vi "大富翁.vi"() -> ()   [LabVIEW 2014] (continued)
                        n2318 = property on="11房1" class="Bool (strict)"("Visible"=TRUE) -> ()  [unwired: 2 in, 2 out]
                      }
                    }
                  }
                  frame 2 {
                    n2319 = flat-sequence {
                      frame #0 {
                        n2320 = local write "11房2"(TRUE ("1房2")) -> ()
                      }
                      frame #1 {
                        n2321 = property on="11房2" class="Bool (strict)"("Visible"=TRUE ("1房2")) -> ()  [unwired: 2 in, 2 out]
                      }
                    }
                  }
                  frame 3 {
                    n2322 = flat-sequence {
                      frame #0 {
                        n2323 = local write "11房3"(TRUE) -> ()
                      }
                      frame #1 {
                        n2324 = property on="11房3" class="Bool (strict)"("Visible"=TRUE) -> ()  [unwired: 2 in, 2 out]
                      }
                    }
                  }
                  frame 4 {
                    n2325 = flat-sequence {
                      frame #0 {
                        n2326 = local write "11房4"(TRUE) -> ()
                      }
                      frame #1 {
                        n2327 = property on="11房4" class="Bool (strict)"("Visible"=TRUE) -> ()  [unwired: 2 in, 2 out]
                      }
                    }
                  }
                  frame 5 {
                    n2328 = flat-sequence {
                      frame #0 {
                        n2329 = local write "11旅1"(TRUE) -> ()
                      }
                      frame #1 {
                        n2330 = property on="11旅1" class="Bool (strict)"("Visible"=TRUE) -> ()  [unwired: 2 in, 2 out]
                      }
                    }
                  }
                  frame 6 {
                    n2331 = flat-sequence {
                      frame #0 {
                        n2332 = local write "11旅2"(TRUE) -> ()
                      }
                      frame #1 {
                        n2333 = property on="11旅2" class="Bool (strict)"("Visible"=TRUE) -> ()  [unwired: 2 in, 2 out]
                      }
                    }
                  }
                  frame 7 {
                    n2334 = flat-sequence {
                      frame #0 {
                        n2335 = local write "11旅3"(TRUE) -> ()
                      }
                      frame #1 {
                        n2336 = property on="11旅3" class="Bool (strict)"("Visible"=TRUE) -> ()  [unwired: 2 in, 2 out]
                      }
                    }
                  }
                  frame 8 {
                    n2337 = flat-sequence {
                      frame #0 {
                        n2338 = local write "11旅4"(TRUE) -> ()
                      }
                      frame #1 {
                        n2339 = property on="11旅4" class="Bool (strict)"("Visible"=TRUE) -> ()  [unwired: 2 in, 2 out]
                      }
                    }
                  }
                }
                n2340 = case shown="1, Default" w1722 {
                  tunnel: w1726 -> [w1758 w1759 w1760 w1761]
                  frame 1, Default {
                    n2341 = local write "玩家一財產"(w1758) -> ()
                  }
                  frame 2 {
                    n2342 = local write "玩家二財產"(w1759) -> ()
                  }
                  frame 3 {
                    n2343 = local write "玩家三財產"(w1760) -> ()
                  }
                  frame 4 {
                    n2344 = local write "玩家四財產"(w1761) -> ()
                  }
                }
              }
              frame True {
                # "無主地"
                n2345 = call "購買土地.vi"() -> ("確定 2"=w1768:bool)  [unwired: 3 in]
                n2346 = case shown="True" w1768 {
                  tunnel: w1767 -> [_ w1772]
                  frame False {
                    # "不買"
                  }
                  frame True {
                    # "要買"
                    n2347 = local read "換誰?"() -> (w1773:dbl)
                    n2348 = case shown="4" w1773 {
                      tunnel: [w1800 w1801 w1802 w1803] -> w1771
                      frame 1, Default {
                        n2349 = local read "玩家一財產"() -> (w1800:dbl)
                      }
                      frame 2 {
                        n2350 = local read "玩家二財產"() -> (w1801:dbl)
                      }
                      frame 3 {
                        n2351 = local read "玩家三財產"() -> (w1802:dbl)
                      }
                      frame 4 {
                        n2352 = local read "玩家四財產"() -> (w1803:dbl)
                      }
                    }
                    n2353 = call "各種價格.vi"("Numeric"=w1772) -> ("買空地"=w1770:dbl)  [unwired: 4 in, 5 out]
                    n2354 = Greater Or Equal?(x=w1771, y=w1770) -> (x >= y?=w1769:bool)
                    n2355 = case shown="True" w1769 {
                      tunnel: w1772 -> [_ w1774]
                      frame False {
                        # "錢不夠"
                        n2356 = call "錢不夠.vi"() -> ()  [unwired: 4 in]
                      }
                      frame True {
                        # "錢夠"
                        n2357 = local read "換誰?"() -> (w1775:dbl)
                        n2358 = case shown="2" w1775 {
                          selector: w1775 -> [w1779 w1785 w1791 w1797]
                          tunnel: w1774 -> [w1778 w1784 w1790 w1796]
                          frame 1, Default {
                            # "誰買了地"
                            n2359 = call "各種價格.vi"("Numeric"=w1778) -> ("買空地"=w1777:dbl)  [unwired: 4 in, 5 out]
                            n2360 = local read "玩家一財產"() -> (w1781:dbl)
                            n2361 = Subtract(x=w1781, y=w1777) -> (x-y=w1780:dbl)
                            n2362 = local write "玩家一財產"(w1780) -> ()
                            n2363 = call "數字轉顏色.vi"("數字"=w1779) -> ("顏色數字"=w1776:dbl)  [unwired: 2 in]
                            n2364 = local write "11蘭嶼"(w1776) -> ()
                            n2365 = local write "蘭嶼所有"(w1776) -> ()
                          }
                          frame 2 {
                            # "誰買了地"
                            n2366 = call "各種價格.vi"("Numeric"=w1784) -> ("買空地"=w1783:dbl)  [unwired: 4 in, 5 out]
                            n2367 = local read "玩家二財產"() -> (w1787:dbl)
                            n2368 = Subtract(x=w1787, y=w1783) -> (x-y=w1786:dbl)
                            n2369 = local write "玩家二財產"(w1786) -> ()
                            n2370 = call "數字轉顏色.vi"("數字"=w1785) -> ("顏色數字"=w1782:dbl)  [unwired: 2 in]
                            n2371 = local write "11蘭嶼"(w1782) -> ()
                            n2372 = local write "蘭嶼所有"(w1782) -> ()
                          }
                          frame 3 {
                            # "誰買了地"
                            n2373 = local read "玩家三財產"() -> (w1792:dbl)
                            n2374 = call "各種價格.vi"("Numeric"=w1790) -> ("買空地"=w1789:dbl)  [unwired: 4 in, 5 out]
                            n2375 = Subtract(x=w1792, y=w1789) -> (x-y=w1793:dbl)
                            n2376 = call "數字轉顏色.vi"("數字"=w1791) -> ("顏色數字"=w1788:dbl)  [unwired: 2 in]
                            n2377 = local write "玩家三財產"(w1793) -> ()
                            n2378 = local write "11蘭嶼"(w1788) -> ()
                            n2379 = local write "蘭嶼所有"(w1788) -> ()
                          }
                          frame 4 {
                            # "誰買了地"
                            n2380 = call "各種價格.vi"("Numeric"=w1796) -> ("買空地"=w1795:dbl)  [unwired: 4 in, 5 out]
                            n2381 = local read "玩家四財產"() -> (w1799:dbl)
                            n2382 = Subtract(x=w1799, y=w1795) -> (x-y=w1798:dbl)
                            n2383 = local write "玩家四財產"(w1798) -> ()
                            n2384 = call "數字轉顏色.vi"("數字"=w1797) -> ("顏色數字"=w1794:dbl)  [unwired: 2 in]
                            n2385 = local write "11蘭嶼"(w1794) -> ()
                            n2386 = local write "蘭嶼所有"(w1794) -> ()
                          }
                        }
                      }
                    }
                  }
                }
              }
            }
          }
          frame 12 {
            n2387 = local read "金門縣所有"() -> (w1804:u32)
            n2388 = Equal?(x=w1804, y=u32 16777215) -> (x = y?=w1807:bool)
            n2389 = case shown="False" w1807 {
              tunnel: w1806 -> [w1830 w1868]
              tunnel: [w1820 FALSE] -> w1805
              frame False {
                # "有主地"
                n2390 = local read "換誰?"() -> (w1823:dbl)
                n2391 = local read "金門縣所有"() -> (w1811:u32)
                n2392 = call "數字轉顏色.vi"("數字"=w1823) -> ("顏色數字"=w1834:dbl)  [unwired: 2 in]
                n2393 = case shown="4" w1823 {
                  tunnel: [w1863 w1864 w1865 w1866] -> w1829
                  frame 1, Default {
                    n2394 = local read "玩家一財產"() -> (w1863:dbl)
                  }
                  frame 2 {
                    n2395 = local read "玩家二財產"() -> (w1864:dbl)
                  }
                  frame 3 {
                    n2396 = local read "玩家三財產"() -> (w1865:dbl)
                  }
                  frame 4 {
                    n2397 = local read "玩家四財產"() -> (w1866:dbl)
                  }
                }
                n2398 = Equal?(x=w1811, y=w1834) -> (x = y?=w1833:bool)
                n2399 = local read "12旅4"() -> (w1819:bool)
                n2400 = local read "12旅3"() -> (w1818:bool)
                n2401 = local read "12旅2"() -> (w1817:bool)
                n2402 = local read "12旅1"() -> (w1816:bool)
                n2403 = local read "12房4"() -> (w1815:bool)
                n2404 = local read "12房3"() -> (w1814:bool)
                n2405 = local read "12房2"() -> (w1813:bool)
                n2406 = local read "12房1"() -> (w1812:bool)
                n2407 = local read "金門縣所有"() -> (w1810:u32)
                n2408 = call "房子數量.vi"("房子 1"=w1812, "房子 2"=w1813, "房子 3"=w1814, "房子 4"=w1815, "旅館 1"=w1816, "旅館 2"=w1817, "旅館 3"=w1818, "旅館 4"=w1819) -> ("房子數"=w1832:dbl, "旅館數"=w1831:dbl)  [unwired: 18 in]
                n2409 = call "顏色轉數字.vi"("顏色數字"=w1810) -> ("數字"=w1821:dbl)  [unwired: 2 in]
                n2410 = case shown="1, Default" w1821 {
                  tunnel: [w1839 w1840 w1841 w1842] -> w1825
                  frame 1, Default {
                    n2411 = local read "玩家一財產"() -> (w1839:dbl)
                  }
                  frame 2 {
                    n2412 = local read "玩家二財產"() -> (w1840:dbl)
                  }
                  frame 3 {
                    n2413 = local read "玩家三財產"() -> (w1841:dbl)
                  }
                  frame 4 {
                    n2414 = local read "玩家四財產"() -> (w1842:dbl)
                  }
                }
                n2415 = call "走到地.vi"("房子數量"=w1832, "自己的地?"=w1833, "旅館數量"=w1831, "編號"=w1830, "走到人財產"=w1829) -> ("走到人-?"=w1828:dbl, "蓋第幾棟"=w1826:dbl, "地主+?"=w1824:dbl, "破產?"=w1820:bool)
                n2416 = Subtract(x=w1829, y=w1828) -> (x-y=w1827:dbl)
                n2417 = Add(x=w1824, y=w1825) -> (x+y=w1822:dbl)
                n2418 = case shown="2" w1821 {
                  tunnel: w1822 -> [w1835 w1836 w1837 w1838]
                  frame 1, Default {
                    n2419 = local write "玩家一財產"(w1835) -> ()
                  }
                  frame 2 {
                    n2420 = local write "玩家二財產"(w1836) -> ()
                  }
                  frame 3 {
                    n2421 = local write "玩家三財產"(w1837) -> ()
                  }
                  frame 4 {
                    n2422 = local write "玩家四財產"(w1838) -> ()
                  }
                }
                n2423 = case shown="2" w1826 {
                  frame 0, Default {
                  }
                  frame 1 {
                    n2424 = flat-sequence {
                      frame #0 {
                        n2425 = local write "12房1"(TRUE ("1房1")) -> ()
                      }
                      frame #1 {
                        n2426 = property on="12房1" class="Bool (strict)"("Visible"=TRUE) -> ()  [unwired: 2 in, 2 out]
                      }
                    }
                  }
                  frame 2 {
                    n2427 = flat-sequence {
                      frame #0 {
                        n2428 = local write "12房2"(TRUE ("1房2")) -> ()
                      }
                      frame #1 {
                        n2429 = property on="12房2" class="Bool (strict)"("Visible"=TRUE ("1房2")) -> ()  [unwired: 2 in, 2 out]
                      }
                    }
                  }
                  frame 3 {
                    n2430 = flat-sequence {
                      frame #0 {
                        n2431 = local write "12房3"(TRUE) -> ()
                      }
                      frame #1 {
                        n2432 = property on="12房3" class="Bool (strict)"("Visible"=TRUE) -> ()  [unwired: 2 in, 2 out]
                      }
                    }
                  }
                  frame 4 {
                    n2433 = flat-sequence {
                      frame #0 {
                        n2434 = local write "12房4"(TRUE) -> ()
                      }
                      frame #1 {
                        n2435 = property on="12房4" class="Bool (strict)"("Visible"=TRUE) -> ()  [unwired: 2 in, 2 out]
                      }
                    }
                  }
                  frame 5 {
                    n2436 = flat-sequence {
                      frame #0 {
                        n2437 = local write "12旅1"(TRUE) -> ()
                      }
                      frame #1 {
                        n2438 = property on="12旅1" class="Bool (strict)"("Visible"=TRUE) -> ()  [unwired: 2 in, 2 out]
                      }
                    }
                  }
                  frame 6 {
                    n2439 = flat-sequence {
                      frame #0 {
                        n2440 = local write "12旅2"(TRUE) -> ()
                      }
                      frame #1 {
                        n2441 = property on="12旅2" class="Bool (strict)"("Visible"=TRUE) -> ()  [unwired: 2 in, 2 out]
                      }
                    }
                  }
                  frame 7 {
                    n2442 = flat-sequence {
                      frame #0 {
                        n2443 = local write "12旅3"(TRUE) -> ()
                      }
                      frame #1 {
                        n2444 = property on="12旅3" class="Bool (strict)"("Visible"=TRUE) -> ()  [unwired: 2 in, 2 out]
                      }
                    }
                  }
                  frame 8 {
                    n2445 = flat-sequence {
                      frame #0 {
                        n2446 = local write "12旅4"(TRUE) -> ()
                      }
                      frame #1 {
                        n2447 = property on="12旅4" class="Bool (strict)"("Visible"=TRUE) -> ()  [unwired: 2 in, 2 out]
                      }
                    }
                  }
                }
                n2448 = case shown="1, Default" w1823 {
                  tunnel: w1827 -> [w1859 w1860 w1861 w1862]
                  frame 1, Default {
                    n2449 = local write "玩家一財產"(w1859) -> ()
                  }
                  frame 2 {
                    n2450 = local write "玩家二財產"(w1860) -> ()
                  }
                  frame 3 {
                    n2451 = local write "玩家三財產"(w1861) -> ()
                  }
                  frame 4 {
                    n2452 = local write "玩家四財產"(w1862) -> ()
                  }
                }
              }
              frame True {
                # "無主地"
                n2453 = call "購買土地.vi"() -> ("確定 2"=w1869:bool)  [unwired: 3 in]
                n2454 = case shown="True" w1869 {
                  tunnel: w1868 -> [_ w1873]
                  frame False {
                    # "不買"
                  }
                  frame True {
                    # "要買"
                    n2455 = local read "換誰?"() -> (w1874:dbl)
                    n2456 = case shown="4" w1874 {
                      tunnel: [w1901 w1902 w1903 w1904] -> w1872
                      frame 1, Default {
                        n2457 = local read "玩家一財產"() -> (w1901:dbl)
                      }
                      frame 2 {
                        n2458 = local read "玩家二財產"() -> (w1902:dbl)
                      }
                      frame 3 {
                        n2459 = local read "玩家三財產"() -> (w1903:dbl)
                      }
                      frame 4 {
                        n2460 = local read "玩家四財產"() -> (w1904:dbl)
                      }
                    }
                    n2461 = call "各種價格.vi"("Numeric"=w1873) -> ("買空地"=w1871:dbl)  [unwired: 4 in, 5 out]
                    n2462 = Greater Or Equal?(x=w1872, y=w1871) -> (x >= y?=w1870:bool)
                    n2463 = case shown="True" w1870 {
                      tunnel: w1873 -> [_ w1875]
                      frame False {
                        # "錢不夠"
                        n2464 = call "錢不夠.vi"() -> ()  [unwired: 4 in]
                      }
                      frame True {
                        # "錢夠"
                        n2465 = local read "換誰?"() -> (w1876:dbl)
                        n2466 = case shown="1, Default" w1876 {
                          selector: w1876 -> [w1880 w1886 w1892 w1898]
                          tunnel: w1875 -> [w1879 w1885 w1891 w1897]
                          frame 1, Default {
                            # "誰買了地"
                            n2467 = call "各種價格.vi"("Numeric"=w1879) -> ("買空地"=w1878:dbl)  [unwired: 4 in, 5 out]
                            n2468 = local read "玩家一財產"() -> (w1882:dbl)
                            n2469 = Subtract(x=w1882, y=w1878) -> (x-y=w1881:dbl)
                            n2470 = local write "玩家一財產"(w1881) -> ()
                            n2471 = call "數字轉顏色.vi"("數字"=w1880) -> ("顏色數字"=w1877:dbl)  [unwired: 2 in]
                            n2472 = local write "12金門"(w1877) -> ()
                            n2473 = local write "金門縣所有"(w1877) -> ()
                          }
                          frame 2 {
                            # "誰買了地"
                            n2474 = call "各種價格.vi"("Numeric"=w1885) -> ("買空地"=w1884:dbl)  [unwired: 4 in, 5 out]
                            n2475 = local read "玩家二財產"() -> (w1888:dbl)
                            n2476 = Subtract(x=w1888, y=w1884) -> (x-y=w1887:dbl)
                            n2477 = local write "玩家二財產"(w1887) -> ()
                            n2478 = call "數字轉顏色.vi"("數字"=w1886) -> ("顏色數字"=w1883:dbl)  [unwired: 2 in]
                            n2479 = local write "12金門"(w1883) -> ()
                            n2480 = local write "金門縣所有"(w1883) -> ()
                          }
                          frame 3 {
                            # "誰買了地"
                            n2481 = local read "玩家三財產"() -> (w1893:dbl)
                            n2482 = call "各種價格.vi"("Numeric"=w1891) -> ("買空地"=w1890:dbl)  [unwired: 4 in, 5 out]
                            n2483 = Subtract(x=w1893, y=w1890) -> (x-y=w1894:dbl)
                            n2484 = call "數字轉顏色.vi"("數字"=w1892) -> ("顏色數字"=w1889:dbl)  [unwired: 2 in]
                            n2485 = local write "玩家三財產"(w1894) -> ()
                            n2486 = local write "12金門"(w1889) -> ()
                            n2487 = local write "金門縣所有"(w1889) -> ()
                          }
                          frame 4 {
                            # "誰買了地"
                            n2488 = call "各種價格.vi"("Numeric"=w1897) -> ("買空地"=w1896:dbl)  [unwired: 4 in, 5 out]
                            n2489 = local read "玩家四財產"() -> (w1900:dbl)
                            n2490 = Subtract(x=w1900, y=w1896) -> (x-y=w1899:dbl)
                            n2491 = local write "玩家四財產"(w1899) -> ()
                            n2492 = call "數字轉顏色.vi"("數字"=w1898) -> ("顏色數字"=w1895:dbl)  [unwired: 2 in]
                            n2493 = local write "12金門"(w1895) -> ()
                            n2494 = local write "金門縣所有"(w1895) -> ()
                          }
                        }
                      }
                    }
                  }
                }
              }
            }
          }
          frame 13 {
            n2495 = call "13監獄.vi"() -> ()  [unwired: 4 in]
          }
          frame 14 {
            n2496 = local read "馬祖所有"() -> (w1907:u32)
            n2497 = Equal?(x=w1907, y=u32 16777215) -> (x = y?=w1910:bool)
            n2498 = case shown="False" w1910 {
              tunnel: w1909 -> [w1933 w1971]
              tunnel: [w1923 FALSE] -> w1908
              frame False {
                # "有主地"
                n2499 = local read "馬祖所有"() -> (w1913:u32)
                n2500 = local read "換誰?"() -> (w1926:dbl)
                n2501 = call "數字轉顏色.vi"("數字"=w1926) -> ("顏色數字"=w1937:dbl)  [unwired: 2 in]
                n2502 = case shown="4" w1926 {
                  tunnel: [w1966 w1967 w1968 w1969] -> w1932
                  frame 1, Default {
                    n2503 = local read "玩家一財產"() -> (w1966:dbl)
                  }
                  frame 2 {
                    n2504 = local read "玩家二財產"() -> (w1967:dbl)
                  }
                  frame 3 {
                    n2505 = local read "玩家三財產"() -> (w1968:dbl)
                  }
                  frame 4 {
                    n2506 = local read "玩家四財產"() -> (w1969:dbl)
                  }
                }
                n2507 = Equal?(x=w1913, y=w1937) -> (x = y?=w1936:bool)
                n2508 = local read "馬祖所有"() -> (w1914:u32)
                n2509 = local read "14旅4"() -> (w1915:bool)
                n2510 = local read "14旅3"() -> (w1916:bool)
                n2511 = local read "14旅2"() -> (w1917:bool)
                n2512 = local read "14旅1"() -> (w1918:bool)
                n2513 = local read "14房4"() -> (w1919:bool)
                n2514 = local read "14房3"() -> (w1920:bool)
                n2515 = local read "14房2"() -> (w1921:bool)
                n2516 = local read "14房1"() -> (w1922:bool)
                n2517 = call "房子數量.vi"("房子 1"=w1922, "房子 2"=w1921, "房子 3"=w1920, "房子 4"=w1919, "旅館 1"=w1918, "旅館 2"=w1917, "旅館 3"=w1916, "旅館 4"=w1915) -> ("房子數"=w1935:dbl, "旅館數"=w1934:dbl)  [unwired: 18 in]
                n2518 = call "顏色轉數字.vi"("顏色數字"=w1914) -> ("數字"=w1924:dbl)  [unwired: 2 in]
                n2519 = case shown="1, Default" w1924 {
                  tunnel: [w1942 w1943 w1944 w1945] -> w1928
                  frame 1, Default {
                    n2520 = local read "玩家一財產"() -> (w1942:dbl)
                  }
                  frame 2 {
                    n2521 = local read "玩家二財產"() -> (w1943:dbl)
                  }
                  frame 3 {
                    n2522 = local read "玩家三財產"() -> (w1944:dbl)
                  }
                  frame 4 {
                    n2523 = local read "玩家四財產"() -> (w1945:dbl)
                  }
                }
                n2524 = call "走到地.vi"("房子數量"=w1935, "自己的地?"=w1936, "旅館數量"=w1934, "編號"=w1933, "走到人財產"=w1932) -> ("走到人-?"=w1931:dbl, "蓋第幾棟"=w1929:dbl, "地主+?"=w1927:dbl, "破產?"=w1923:bool)
                n2525 = Subtract(x=w1932, y=w1931) -> (x-y=w1930:dbl)
                n2526 = Add(x=w1927, y=w1928) -> (x+y=w1925:dbl)
                n2527 = case shown="1, Default" w1924 {
                  tunnel: w1925 -> [w1938 w1939 w1940 w1941]
                  frame 1, Default {
                    n2528 = local write "玩家一財產"(w1938) -> ()
                  }
                  frame 2 {
                    n2529 = local write "玩家二財產"(w1939) -> ()
                  }
                  frame 3 {
                    n2530 = local write "玩家三財產"(w1940) -> ()
                  }
                  frame 4 {
                    n2531 = local write "玩家四財產"(w1941) -> ()
                  }
                }
                n2532 = case shown="8" w1929 {
                  frame 0, Default {
                  }
                  frame 1 {
                    n2533 = flat-sequence {
                      frame #0 {
                        n2534 = local write "14房1"(TRUE ("1房1")) -> ()
                      }
                      frame #1 {
                        n2535 = property on="14房1" class="Bool (strict)"("Visible"=TRUE) -> ()  [unwired: 2 in, 2 out]
                      }
                    }
                  }
                  frame 2 {
                    n2536 = flat-sequence {
                      frame #0 {
                        n2537 = local write "14房2"(TRUE ("1房2")) -> ()
                      }
                      frame #1 {
                        n2538 = property on="14房2" class="Bool (strict)"("Visible"=TRUE ("1房2")) -> ()  [unwired: 2 in, 2 out]
                      }
                    }
                  }
                  frame 3 {
                    n2539 = flat-sequence {
                      frame #0 {
                        n2540 = local write "14房3"(TRUE) -> ()
                      }
                      frame #1 {
                        n2541 = property on="14房3" class="Bool (strict)"("Visible"=TRUE) -> ()  [unwired: 2 in, 2 out]
                      }
                    }
                  }
                  frame 4 {
                    n2542 = flat-sequence {
                      frame #0 {
                        n2543 = local write "14房4"(TRUE) -> ()
                      }
                      frame #1 {
                        n2544 = property on="14房4" class="Bool (strict)"("Visible"=TRUE) -> ()  [unwired: 2 in, 2 out]
                      }
                    }
                  }
                  frame 5 {
                    n2545 = flat-sequence {
                      frame #0 {
                        n2546 = local write "14旅1"(TRUE) -> ()
                      }
                      frame #1 {
                        n2547 = property on="14旅1" class="Bool (strict)"("Visible"=TRUE) -> ()  [unwired: 2 in, 2 out]
                      }
                    }
                  }
                  frame 6 {
                    n2548 = flat-sequence {
                      frame #0 {
                        n2549 = local write "14旅2"(TRUE) -> ()
                      }
                      frame #1 {
                        n2550 = property on="14旅2" class="Bool (strict)"("Visible"=TRUE) -> ()  [unwired: 2 in, 2 out]
                      }
                    }
                  }
                  frame 7 {
                    n2551 = flat-sequence {
                      frame #0 {
                        n2552 = local write "14旅3"(TRUE) -> ()
                      }
                      frame #1 {
                        n2553 = property on="14旅3" class="Bool (strict)"("Visible"=TRUE) -> ()  [unwired: 2 in, 2 out]
                      }
                    }
                  }
                  frame 8 {
                    n2554 = flat-sequence {
                      frame #0 {
                        n2555 = local write "14旅4"(TRUE) -> ()
                      }
                      frame #1 {
                        n2556 = property on="14旅4" class="Bool (strict)"("Visible"=TRUE) -> ()  [unwired: 2 in, 2 out]
                      }
                    }
                  }
                }
                n2557 = case shown="1, Default" w1926 {
                  tunnel: w1930 -> [w1962 w1963 w1964 w1965]
                  frame 1, Default {
                    n2558 = local write "玩家一財產"(w1962) -> ()
                  }
                  frame 2 {
                    n2559 = local write "玩家二財產"(w1963) -> ()
                  }
                  frame 3 {
                    n2560 = local write "玩家三財產"(w1964) -> ()
                  }
                  frame 4 {
                    n2561 = local write "玩家四財產"(w1965) -> ()
                  }
                }
              }
              frame True {
                # "無主地"
                n2562 = call "購買土地.vi"() -> ("確定 2"=w1972:bool)  [unwired: 3 in]
                n2563 = case shown="True" w1972 {
                  tunnel: w1971 -> [_ w1976]
                  frame False {
                    # "不買"
                  }
                  frame True {
                    # "要買"
                    n2564 = local read "換誰?"() -> (w1977:dbl)
                    n2565 = case shown="4" w1977 {
                      tunnel: [w2004 w2005 w2006 w2007] -> w1975
                      frame 1, Default {
                        n2566 = local read "玩家一財產"() -> (w2004:dbl)
                      }
                      frame 2 {
                        n2567 = local read "玩家二財產"() -> (w2005:dbl)
                      }
                      frame 3 {
                        n2568 = local read "玩家三財產"() -> (w2006:dbl)
                      }
                      frame 4 {
                        n2569 = local read "玩家四財產"() -> (w2007:dbl)
                      }
                    }
                    n2570 = call "各種價格.vi"("Numeric"=w1976) -> ("買空地"=w1974:dbl)  [unwired: 4 in, 5 out]
                    n2571 = Greater Or Equal?(x=w1975, y=w1974) -> (x >= y?=w1973:bool)
                    n2572 = case shown="True" w1973 {
                      tunnel: w1976 -> [_ w1978]
                      frame False {
                        # "錢不夠"
                        n2573 = call "錢不夠.vi"() -> ()  [unwired: 4 in]
                      }
                      frame True {
                        # "錢夠"
                        n2574 = local read "換誰?"() -> (w1979:dbl)
                        n2575 = case shown="2" w1979 {
                          selector: w1979 -> [w1983 w1989 w1995 w2001]
                          tunnel: w1978 -> [w1982 w1988 w1994 w2000]
                          frame 1, Default {
                            # "誰買了地"
                            n2576 = call "各種價格.vi"("Numeric"=w1982) -> ("買空地"=w1981:dbl)  [unwired: 4 in, 5 out]
                            n2577 = local read "玩家一財產"() -> (w1985:dbl)
                            n2578 = Subtract(x=w1985, y=w1981) -> (x-y=w1984:dbl)
                            n2579 = local write "玩家一財產"(w1984) -> ()
                            n2580 = call "數字轉顏色.vi"("數字"=w1983) -> ("顏色數字"=w1980:dbl)  [unwired: 2 in]
                            n2581 = local write "馬祖所有"(w1980) -> ()
                            n2582 = local write "14馬祖"(w1980) -> ()
                          }
                          frame 2 {
                            # "誰買了地"
                            n2583 = call "各種價格.vi"("Numeric"=w1988) -> ("買空地"=w1987:dbl)  [unwired: 4 in, 5 out]
                            n2584 = local read "玩家二財產"() -> (w1991:dbl)
                            n2585 = Subtract(x=w1991, y=w1987) -> (x-y=w1990:dbl)
                            n2586 = local write "玩家二財產"(w1990) -> ()
                            n2587 = call "數字轉顏色.vi"("數字"=w1989) -> ("顏色數字"=w1986:dbl)  [unwired: 2 in]
                            n2588 = local write "馬祖所有"(w1986) -> ()
                            n2589 = local write "14馬祖"(w1986) -> ()
                          }
                          frame 3 {
                            # "誰買了地"
                            n2590 = local read "玩家三財產"() -> (w1996:dbl)
                            n2591 = call "各種價格.vi"("Numeric"=w1994) -> ("買空地"=w1993:dbl)  [unwired: 4 in, 5 out]
                            n2592 = Subtract(x=w1996, y=w1993) -> (x-y=w1997:dbl)
                            n2593 = call "數字轉顏色.vi"("數字"=w1995) -> ("顏色數字"=w1992:dbl)  [unwired: 2 in]
                            n2594 = local write "玩家三財產"(w1997) -> ()
                            n2595 = local write "馬祖所有"(w1992) -> ()
                            n2596 = local write "14馬祖"(w1992) -> ()
                          }
                          frame 4 {
                            # "誰買了地"
                            n2597 = call "各種價格.vi"("Numeric"=w2000) -> ("買空地"=w1999:dbl)  [unwired: 4 in, 5 out]
                            n2598 = local read "玩家四財產"() -> (w2003:dbl)
                            n2599 = Subtract(x=w2003, y=w1999) -> (x-y=w2002:dbl)
                            n2600 = local write "玩家四財產"(w2002) -> ()
                            n2601 = call "數字轉顏色.vi"("數字"=w2001) -> ("顏色數字"=w1998:dbl)  [unwired: 2 in]
                            n2602 = local write "馬祖所有"(w1998) -> ()
                            n2603 = local write "14馬祖"(w1998) -> ()
                          }
                        }
                      }
                    }
                  }
                }
              }
            }
          }
          frame 15 {
            n2604 = local read "小琉球所有"() -> (w2008:u32)
            n2605 = Equal?(x=w2008, y=u32 16777215) -> (x = y?=w2011:bool)
            n2606 = case shown="False" w2011 {
              tunnel: w2009 -> [w2034 w2072]
              tunnel: [w2024 FALSE] -> w2010
              frame False {
                # "有主地"
                n2607 = local read "換誰?"() -> (w2027:dbl)
                n2608 = local read "小琉球所有"() -> (w2015:u32)
                n2609 = call "數字轉顏色.vi"("數字"=w2027) -> ("顏色數字"=w2038:dbl)  [unwired: 2 in]
                n2610 = local read "小琉球所有"() -> (w2014:u32)
                n2611 = case shown="3" w2027 {
                  tunnel: [w2067 w2068 w2069 w2070] -> w2033
                  frame 1, Default {
                    n2612 = local read "玩家一財產"() -> (w2067:dbl)
                  }
                  frame 2 {
                    n2613 = local read "玩家二財產"() -> (w2068:dbl)
                  }
                  frame 3 {
                    n2614 = local read "玩家三財產"() -> (w2069:dbl)
                  }
                  frame 4 {
                    n2615 = local read "玩家四財產"() -> (w2070:dbl)
                  }
                }
                n2616 = Equal?(x=w2015, y=w2038) -> (x = y?=w2037:bool)
                n2617 = local read "15旅4"() -> (w2016:bool)
                n2618 = local read "15旅3"() -> (w2017:bool)
                n2619 = local read "15旅2"() -> (w2018:bool)
                n2620 = local read "15旅1"() -> (w2019:bool)
                n2621 = local read "15房4"() -> (w2020:bool)
                n2622 = local read "15房3"() -> (w2021:bool)
                n2623 = local read "15房2"() -> (w2022:bool)
                n2624 = local read "15房1"() -> (w2023:bool)
                n2625 = call "房子數量.vi"("房子 1"=w2023, "房子 2"=w2022, "房子 3"=w2021, "房子 4"=w2020, "旅館 1"=w2019, "旅館 2"=w2018, "旅館 3"=w2017, "旅館 4"=w2016) -> ("房子數"=w2036:dbl, "旅館數"=w2035:dbl)  [unwired: 18 in]
                n2626 = call "顏色轉數字.vi"("顏色數字"=w2014) -> ("數字"=w2025:dbl)  [unwired: 2 in]
                n2627 = case shown="1, Default" w2025 {
                  tunnel: [w2043 w2044 w2045 w2046] -> w2029
                  frame 1, Default {
                    n2628 = local read "玩家一財產"() -> (w2043:dbl)
                  }
                  frame 2 {
                    n2629 = local read "玩家二財產"() -> (w2044:dbl)
                  }
                  frame 3 {
                    n2630 = local read "玩家三財產"() -> (w2045:dbl)
                  }
                  frame 4 {
                    n2631 = local read "玩家四財產"() -> (w2046:dbl)
                  }
                }
                n2632 = call "走到地.vi"("房子數量"=w2036, "自己的地?"=w2037, "旅館數量"=w2035, "編號"=w2034, "走到人財產"=w2033) -> ("走到人-?"=w2032:dbl, "蓋第幾棟"=w2030:dbl, "地主+?"=w2028:dbl, "破產?"=w2024:bool)
                n2633 = Subtract(x=w2033, y=w2032) -> (x-y=w2031:dbl)
                n2634 = Add(x=w2028, y=w2029) -> (x+y=w2026:dbl)
                n2635 = case shown="1, Default" w2025 {
                  tunnel: w2026 -> [w2039 w2040 w2041 w2042]
                  frame 1, Default {
                    n2636 = local write "玩家一財產"(w2039) -> ()
                  }
                  frame 2 {
                    n2637 = local write "玩家二財產"(w2040) -> ()
                  }
                  frame 3 {
                    n2638 = local write "玩家三財產"(w2041) -> ()
                  }
                  frame 4 {
                    n2639 = local write "玩家四財產"(w2042) -> ()
                  }
                }
                n2640 = case shown="8" w2030 {
                  frame 0, Default {
                  }
                  frame 1 {
                    n2641 = flat-sequence {
                      frame #0 {
                        n2642 = local write "15房1"(TRUE ("1房1")) -> ()
                      }
                      frame #1 {
                        n2643 = property on="15房1" class="Bool (strict)"("Visible"=TRUE) -> ()  [unwired: 2 in, 2 out]
                      }
                    }
                  }
                  frame 2 {
                    n2644 = flat-sequence {
                      frame #0 {
                        n2645 = local write "15房2"(TRUE ("1房2")) -> ()
                      }
                      frame #1 {
                        n2646 = property on="15房2" class="Bool (strict)"("Visible"=TRUE ("1房2")) -> ()  [unwired: 2 in, 2 out]
                      }
                    }
                  }
                  frame 3 {
                    n2647 = flat-sequence {
                      frame #0 {
                        n2648 = local write "15房3"(TRUE) -> ()
                      }
                      frame #1 {
                        n2649 = property on="15房3" class="Bool (strict)"("Visible"=TRUE) -> ()  [unwired: 2 in, 2 out]
                      }
                    }
                  }
                  frame 4 {
                    n2650 = flat-sequence {
                      frame #0 {
                        n2651 = local write "15房4"(TRUE) -> ()
                      }
                      frame #1 {
                        n2652 = property on="15房4" class="Bool (strict)"("Visible"=TRUE) -> ()  [unwired: 2 in, 2 out]
                      }
                    }
                  }
                  frame 5 {
                    n2653 = flat-sequence {
                      frame #0 {
                        n2654 = local write "15旅1"(TRUE) -> ()
                      }
                      frame #1 {
                        n2655 = property on="15旅1" class="Bool (strict)"("Visible"=TRUE) -> ()  [unwired: 2 in, 2 out]
                      }
                    }
                  }
                  frame 6 {
                    n2656 = flat-sequence {
                      frame #0 {
                        n2657 = local write "15旅2"(TRUE) -> ()
                      }
                      frame #1 {
                        n2658 = property on="15旅2" class="Bool (strict)"("Visible"=TRUE) -> ()  [unwired: 2 in, 2 out]
                      }
                    }
                  }
                  frame 7 {
                    n2659 = flat-sequence {
                      frame #0 {
                        n2660 = local write "15旅3"(TRUE) -> ()
                      }
                      frame #1 {
                        n2661 = property on="15旅3" class="Bool (strict)"("Visible"=TRUE) -> ()  [unwired: 2 in, 2 out]
                      }
                    }
                  }
                  frame 8 {
                    n2662 = flat-sequence {
                      frame #0 {
                        n2663 = local write "15旅4"(TRUE) -> ()
                      }
                      frame #1 {
                        n2664 = property on="15旅4" class="Bool (strict)"("Visible"=TRUE) -> ()  [unwired: 2 in, 2 out]
                      }
                    }
                  }
                }
                n2665 = case shown="2" w2027 {
                  tunnel: w2031 -> [w2063 w2064 w2065 w2066]
                  frame 1, Default {
                    n2666 = local write "玩家一財產"(w2063) -> ()
                  }
                  frame 2 {
                    n2667 = local write "玩家二財產"(w2064) -> ()
                  }
                  frame 3 {
                    n2668 = local write "玩家三財產"(w2065) -> ()
                  }
                  frame 4 {
                    n2669 = local write "玩家四財產"(w2066) -> ()
                  }
                }
              }
              frame True {
                # "無主地"
                n2670 = call "購買土地.vi"() -> ("確定 2"=w2073:bool)  [unwired: 3 in]
                n2671 = case shown="True" w2073 {
                  tunnel: w2072 -> [_ w2077]
                  frame False {
                    # "不買"
                  }
                  frame True {
                    # "要買"
                    n2672 = local read "換誰?"() -> (w2078:dbl)
                    n2673 = case shown="4" w2078 {
                      tunnel: [w2105 w2106 w2107 w2108] -> w2076
                      frame 1, Default {
                        n2674 = local read "玩家一財產"() -> (w2105:dbl)
                      }
                      frame 2 {
                        n2675 = local read "玩家二財產"() -> (w2106:dbl)
                      }
                      frame 3 {
                        n2676 = local read "玩家三財產"() -> (w2107:dbl)
                      }
                      frame 4 {
                        n2677 = local read "玩家四財產"() -> (w2108:dbl)
                      }
                    }
                    n2678 = call "各種價格.vi"("Numeric"=w2077) -> ("買空地"=w2075:dbl)  [unwired: 4 in, 5 out]
                    n2679 = Greater Or Equal?(x=w2076, y=w2075) -> (x >= y?=w2074:bool)
                    n2680 = case shown="True" w2074 {
                      tunnel: w2077 -> [_ w2079]
                      frame False {
                        # "錢不夠"
                        n2681 = call "錢不夠.vi"() -> ()  [unwired: 4 in]
                      }
                      frame True {
                        # "錢夠"
                        n2682 = local read "換誰?"() -> (w2080:dbl)
                        n2683 = case shown="1, Default" w2080 {
                          selector: w2080 -> [w2084 w2090 w2096 w2102]
                          tunnel: w2079 -> [w2083 w2089 w2095 w2101]
                          frame 1, Default {
                            # "誰買了地"
                            n2684 = call "各種價格.vi"("Numeric"=w2083) -> ("買空地"=w2082:dbl)  [unwired: 4 in, 5 out]
                            n2685 = local read "玩家一財產"() -> (w2086:dbl)
                            n2686 = Subtract(x=w2086, y=w2082) -> (x-y=w2085:dbl)
                            n2687 = local write "玩家一財產"(w2085) -> ()
                            n2688 = call "數字轉顏色.vi"("數字"=w2084) -> ("顏色數字"=w2081:dbl)  [unwired: 2 in]
                            n2689 = local write "15小琉球"(w2081) -> ()
                            n2690 = local write "小琉球所有"(w2081) -> ()
                          }
                          frame 2 {
                            # "誰買了地"
                            n2691 = call "各種價格.vi"("Numeric"=w2089) -> ("買空地"=w2088:dbl)  [unwired: 4 in, 5 out]
                            n2692 = local read "玩家二財產"() -> (w2092:dbl)
                            n2693 = Subtract(x=w2092, y=w2088) -> (x-y=w2091:dbl)
                            n2694 = local write "玩家二財產"(w2091) -> ()
                            n2695 = call "數字轉顏色.vi"("數字"=w2090) -> ("顏色數字"=w2087:dbl)  [unwired: 2 in]
                            n2696 = local write "15小琉球"(w2087) -> ()
                            n2697 = local write "小琉球所有"(w2087) -> ()
                          }
                          frame 3 {
                            # "誰買了地"
                            n2698 = local read "玩家三財產"() -> (w2097:dbl)
                            n2699 = call "各種價格.vi"("Numeric"=w2095) -> ("買空地"=w2094:dbl)  [unwired: 4 in, 5 out]
                            n2700 = Subtract(x=w2097, y=w2094) -> (x-y=w2098:dbl)
                            n2701 = call "數字轉顏色.vi"("數字"=w2096) -> ("顏色數字"=w2093:dbl)  [unwired: 2 in]
                            n2702 = local write "玩家三財產"(w2098) -> ()
                            n2703 = local write "15小琉球"(w2093) -> ()
                            n2704 = local write "小琉球所有"(w2093) -> ()
                          }
                          frame 4 {
                            # "誰買了地"
                            n2705 = call "各種價格.vi"("Numeric"=w2101) -> ("買空地"=w2100:dbl)  [unwired: 4 in, 5 out]
                            n2706 = local read "玩家四財產"() -> (w2104:dbl)
                            n2707 = Subtract(x=w2104, y=w2100) -> (x-y=w2103:dbl)
                            n2708 = local write "玩家四財產"(w2103) -> ()
                            n2709 = call "數字轉顏色.vi"("數字"=w2102) -> ("顏色數字"=w2099:dbl)  [unwired: 2 in]
                            n2710 = local write "15小琉球"(w2099) -> ()
                            n2711 = local write "小琉球所有"(w2099) -> ()
                          }
                        }
                      }
                    }
                  }
                }
              }
            }
          }
          frame 17 {
            n2712 = local read "墾丁所有"() -> (w2109:u32)
            n2713 = Equal?(x=w2109, y=u32 16777215) -> (x = y?=w2112:bool)
            n2714 = case shown="False" w2112 {
              tunnel: w2110 -> [w2135 w2173]
              tunnel: [w2125 FALSE] -> w2111
              frame False {
                # "有主地"
                n2715 = local read "換誰?"() -> (w2128:dbl)
                n2716 = local read "墾丁所有"() -> (w2116:u32)
                n2717 = call "數字轉顏色.vi"("數字"=w2128) -> ("顏色數字"=w2139:dbl)  [unwired: 2 in]
                n2718 = case shown="4" w2128 {
                  tunnel: [w2168 w2169 w2170 w2171] -> w2134
                  frame 1, Default {
                    n2719 = local read "玩家一財產"() -> (w2168:dbl)
                  }
                  frame 2 {
                    n2720 = local read "玩家二財產"() -> (w2169:dbl)
                  }
                  frame 3 {
                    n2721 = local read "玩家三財產"() -> (w2170:dbl)
                  }
                  frame 4 {
                    n2722 = local read "玩家四財產"() -> (w2171:dbl)
                  }
                }
                n2723 = Equal?(x=w2116, y=w2139) -> (x = y?=w2138:bool)
                n2724 = local read "墾丁所有"() -> (w2115:u32)
                n2725 = local read "17旅4"() -> (w2117:bool)
                n2726 = local read "17旅3"() -> (w2118:bool)
                n2727 = local read "17旅2"() -> (w2119:bool)
                n2728 = local read "17旅1"() -> (w2120:bool)
                n2729 = local read "17房4"() -> (w2121:bool)
                n2730 = local read "17房3"() -> (w2122:bool)
                n2731 = local read "17房2"() -> (w2123:bool)
                n2732 = local read "17房1"() -> (w2124:bool)
                n2733 = call "房子數量.vi"("房子 1"=w2124, "房子 2"=w2123, "房子 3"=w2122, "房子 4"=w2121, "旅館 1"=w2120, "旅館 2"=w2119, "旅館 3"=w2118, "旅館 4"=w2117) -> ("房子數"=w2137:dbl, "旅館數"=w2136:dbl)  [unwired: 18 in]
                n2734 = call "顏色轉數字.vi"("顏色數字"=w2115) -> ("數字"=w2126:dbl)  [unwired: 2 in]
                n2735 = case shown="1, Default" w2126 {
                  tunnel: [w2144 w2145 w2146 w2147] -> w2130
                  frame 1, Default {
                    n2736 = local read "玩家一財產"() -> (w2144:dbl)
                  }
                  frame 2 {
                    n2737 = local read "玩家二財產"() -> (w2145:dbl)
                  }
                  frame 3 {
                    n2738 = local read "玩家三財產"() -> (w2146:dbl)
                  }
                  frame 4 {
                    n2739 = local read "玩家四財產"() -> (w2147:dbl)
                  }
                }
                n2740 = call "走到地.vi"("房子數量"=w2137, "自己的地?"=w2138, "旅館數量"=w2136, "編號"=w2135, "走到人財產"=w2134) -> ("走到人-?"=w2133:dbl, "蓋第幾棟"=w2131:dbl, "地主+?"=w2129:dbl, "破產?"=w2125:bool)
                n2741 = Subtract(x=w2134, y=w2133) -> (x-y=w2132:dbl)
                n2742 = Add(x=w2129, y=w2130) -> (x+y=w2127:dbl)
                n2743 = case shown="1, Default" w2126 {
                  tunnel: w2127 -> [w2140 w2141 w2142 w2143]
                  frame 1, Default {
                    n2744 = local write "玩家一財產"(w2140) -> ()
                  }
                  frame 2 {
                    n2745 = local write "玩家二財產"(w2141) -> ()
                  }
                  frame 3 {
                    n2746 = local write "玩家三財產"(w2142) -> ()
                  }
                  frame 4 {
                    n2747 = local write "玩家四財產"(w2143) -> ()
                  }
                }
                n2748 = case shown="1" w2131 {
                  frame 0, Default {
                  }
                  frame 1 {
                    n2749 = flat-sequence {
                      frame #0 {
                        n2750 = local write "17房1"(TRUE ("1房1")) -> ()
                      }
                      frame #1 {
                        n2751 = property on="17房1" class="Bool (strict)"("Visible"=TRUE) -> ()  [unwired: 2 in, 2 out]
                      }
                    }
                  }
                  frame 2 {
                    n2752 = flat-sequence {
                      frame #0 {
                        n2753 = local write "17房2"(TRUE ("1房2")) -> ()
                      }
                      frame #1 {
                        n2754 = property on="17房2" class="Bool (strict)"("Visible"=TRUE ("1房2")) -> ()  [unwired: 2 in, 2 out]
                      }
                    }
                  }
                  frame 3 {
                    n2755 = flat-sequence {
                      frame #0 {
                        n2756 = local write "17房3"(TRUE) -> ()
                      }
                      frame #1 {
                        n2757 = property on="17房3" class="Bool (strict)"("Visible"=TRUE) -> ()  [unwired: 2 in, 2 out]
                      }
                    }
                  }
                  frame 4 {
                    n2758 = flat-sequence {
                      frame #0 {
                        n2759 = local write "17房4"(TRUE) -> ()
                      }
                      frame #1 {
                        n2760 = property on="17房4" class="Bool (strict)"("Visible"=TRUE) -> ()  [unwired: 2 in, 2 out]
                      }
                    }
                  }
                  frame 5 {
                    n2761 = flat-sequence {
                      frame #0 {
                        n2762 = local write "17旅1"(TRUE) -> ()
                      }
                      frame #1 {
                        n2763 = property on="17旅1" class="Bool (strict)"("Visible"=TRUE) -> ()  [unwired: 2 in, 2 out]
                      }
                    }
                  }
                  frame 6 {
                    n2764 = flat-sequence {
                      frame #0 {
                        n2765 = local write "17旅2"(TRUE) -> ()
                      }
                      frame #1 {
                        n2766 = property on="17旅2" class="Bool (strict)"("Visible"=TRUE) -> ()  [unwired: 2 in, 2 out]
                      }
                    }
                  }
                  frame 7 {
                    n2767 = flat-sequence {
                      frame #0 {
                        n2768 = local write "17旅3"(TRUE) -> ()
                      }
                      frame #1 {
                        n2769 = property on="17旅3" class="Bool (strict)"("Visible"=TRUE) -> ()  [unwired: 2 in, 2 out]
                      }
                    }
                  }
                  frame 8 {
                    n2770 = flat-sequence {
                      frame #0 {
                        n2771 = local write "17旅4"(TRUE) -> ()
                      }
                      frame #1 {
                        n2772 = property on="17旅4" class="Bool (strict)"("Visible"=TRUE) -> ()  [unwired: 2 in, 2 out]
                      }
                    }
                  }
                }
                n2773 = case shown="1, Default" w2128 {
                  tunnel: w2132 -> [w2164 w2165 w2166 w2167]
                  frame 1, Default {
                    n2774 = local write "玩家一財產"(w2164) -> ()
                  }
                  frame 2 {
                    n2775 = local write "玩家二財產"(w2165) -> ()
                  }
                  frame 3 {
                    n2776 = local write "玩家三財產"(w2166) -> ()
                  }
                  frame 4 {
                    n2777 = local write "玩家四財產"(w2167) -> ()
                  }
                }
              }
              frame True {
                # "無主地"
                n2778 = call "購買土地.vi"() -> ("確定 2"=w2174:bool)  [unwired: 3 in]
                n2779 = case shown="False" w2174 {
                  tunnel: w2173 -> [_ w2178]
                  frame False {
                    # "不買"
                  }
                  frame True {
                    # "要買"
                    n2780 = local read "換誰?"() -> (w2179:dbl)
                    n2781 = case shown="4" w2179 {
                      tunnel: [w2206 w2207 w2208 w2209] -> w2177
                      frame 1, Default {
                        n2782 = local read "玩家一財產"() -> (w2206:dbl)
                      }
                      frame 2 {
                        n2783 = local read "玩家二財產"() -> (w2207:dbl)
                      }
                      frame 3 {
                        n2784 = local read "玩家三財產"() -> (w2208:dbl)
                      }
